vi "Get Selected Palette's Color Array.vi"(9 "Selected Palette":string, 11 "Palette Specifications":T1[](array[typedef])) -> (0 "Found?":bool, 3 "Palette Colors":u32[](array[numeric]))   [LabVIEW 2021, in "Palette.lvlib"]
uses:
  Palette.lvlib
  Color Brewer Palette.ctl
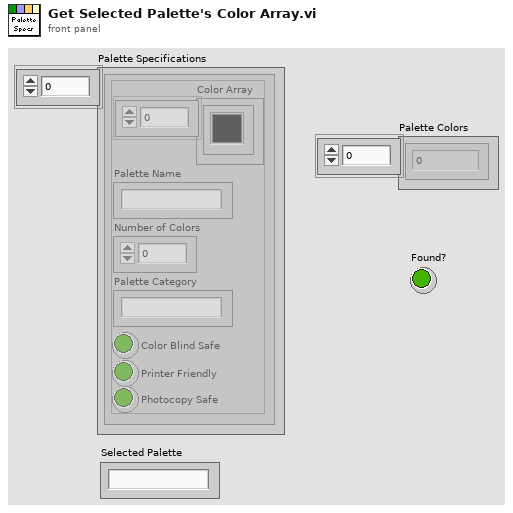
[diagram p1: front panel]
types:
  T1 = typedef "Palette.lvlib/Color Brewer Palette.ctl" = cluster{"Color Array":u32[], "Palette Name":string, "Number of Colors":i32, "Palette Category":string, "Color Blind Safe":bool, "Printer Friendly":bool, "Photocopy Safe":bool}
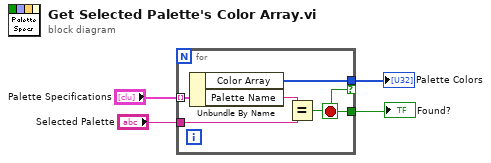
[diagram p0: block diagram]
diagram:
  n1 = for {
    tunnel: "Palette Specifications" -> [w7] mode=indexing
    tunnel: "Selected Palette" -> [w8]
    tunnel: [w6] -> w2 if=w5
    tunnel: [w5] -> w1
    stop <- w5 stop-if-true
    n2 = Unbundle By Name(w7) -> ("Color Array"=w6:u32[], "Palette Name"=w9:string)
    n3 = Equal?(x=w9, y=w8) -> (x = y?=w5:bool)
  }
  "Palette Colors" <- w2
  "Found?" <- w1
